vi "Periodic Tasks V.3.0.vi"(8 "error in":errorcluster) -> ()   [LabVIEW 2017]
doc: "This VI runs in parallel to other tasks. It can contain as many user-defined periodic loops as you need. These can carry out PID or other sorts of timed response."
uses:
  <vilib>/Rock Robotics/WPI/Solenoid/WPI_SolenoidValue.ctl
  <vilib>/Rock Robotics/WPI/DriverStation/WPI_DriverStationRobotMode2.ctl
  Public/Documents/Cross The Road Electronics/Phoenix-LabVIEW/Motor Controller/Get/CTRE_Phoenix_MotorController_GetQuadratureData.vi
  <vilib>/Rock Robotics/Network Tables/NT Read Boolean.vi
  Robot Global Data V.3.0.vi
  <vilib>/Rock Robotics/WPI/Utilities/WPI_GetSetVariantRefNum.vi
  <vilib>/addons/control/pid/pid.llb/PID (DBL).vi
  <vilib>/Rock Robotics/WPI/Solenoid/WPI_SolenoidSetEnum.vi
  <vilib>/Rock Robotics/WPI/RobotDrive/WPI_RobotDriveArcadeDrive_Standard(NoSaturation).vi
  <vilib>/addons/control/pid/NI_PID_pid.lvlib
panel:
  out "Right Intake Motor":dbl
  out "Left Intake Motor":dbl
  out "Read Drive Run Speed":dbl
  out "Collector and Drive Loop Run Speed":dbl
  out "Waveform Chart":T1(graph)
  in  "output range":cluster{"output high":dbl, "output low":dbl}={"output high"=100.0, "output low"=-100.0} {"output low" format="%.2f"; "output high" format="%.2f"}
  in  "PID gains":T2={"proportional gain (Kc)"=1.0, "integral time (Ti, min)"=0.01, "derivative time (Td, min)"=0.0}
  out "Compressor Run Speed":dbl
  out "Error Loop Run Speed":dbl
  out "Right Dart Run Speed":dbl
  out "Left Dart Run Speed":dbl
  out "Read Stuff Run Speed":dbl
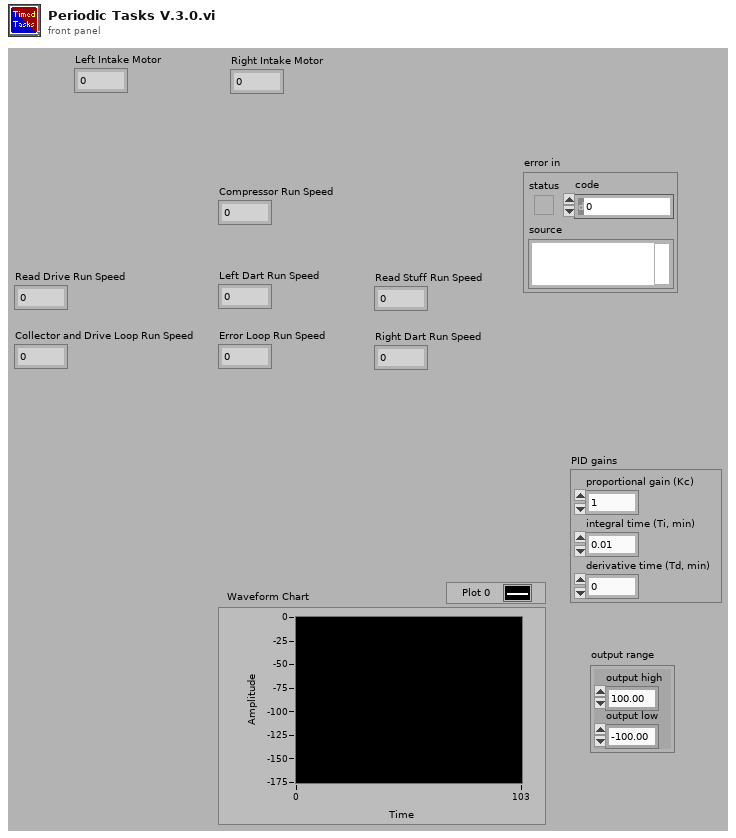
[diagram p1: front panel]
types:
  T1 = cluster{"Collector Angle Motor Wanted Angle":dbl, "Collector Angle Motor Actual Angle":dbl}
  T2 = cluster{"proportional gain (Kc)":dbl, "integral time (Ti, min)":dbl, "derivative time (Td, min)":dbl}
  T3 = cluster{"Pot. Voltage":dbl[], "Corresponding Inches":dbl[]}
  T4 = typedef "WPI_RobotDriveDevRef.ctl" = cluster{"DevStatus":errorcluster, "Motors[]":T5[], "Square Inputs":bool, "Max Output":dbl}
  T5 = typedef "WPI_MotorControlDeviceRef.ctl" = cluster{"DeviceStatus":errorcluster, "Type":T6, "PWM":cluster{"PWM Channel":T7, "DeadBand":T8}, "CAN":cluster{"Device Number":u8, "SetOutput VI Ref":variant, "GetOutput VI Ref":variant, "Enable VI Ref":variant, "Disable VI Ref":variant, "Data":variant}, "Invert":bool, "DIO PWM":cluster{"PWM \"Enable\" Channel":T7, "DIOChannel":T9, "PWM Rate":dbl}}
  T6 = typedef "WPI_MotorControlType.ctl" = enum16{"PWM", "CAN", "DIO PWM"}
  T7 = typedef "FPGA_DIOPWMChannel.ctl" = enum8{"PWM 0", "PWM 1", "PWM 2", "PWM 3", "PWM 4", "PWM 5", "PWM 6", "PWM 7", "PWM 8", "PWM 9", "PWM MXP 0", "PWM MXP 1", "PWM MXP 2", "PWM MXP 3", "PWM MXP 4", "PWM MXP 5", "PWM MXP 6", "PWM MXP 7", "PWM MXP 8", "PWM MXP 9", "Invalid"}
  T8 = typedef "WPI_PWMDeadband.ctl" = cluster{"Name":string, "maxPositivePwm":i32, "minPositivePwm":i32, "centerPwm":i32, "maxNegativePwm":i32, "minNegativePwm":i32, "angularRange":u16}
  T9 = typedef "FPGA_DIOChannel.ctl" = enum8{"DIO 0", "DIO 1", "DIO 2", "DIO 3", "DIO 4", "DIO 5", "DIO 6", "DIO 7", "DIO 8", "DIO 9", "DIO MXP 0", "DIO MXP 1", "DIO MXP 2", "DIO MXP 3", "DIO MXP 4", "DIO MXP 5", "DIO MXP 6", "DIO MXP 7", "DIO MXP 8", "DIO MXP 9", "DIO MXP 10", "DIO MXP 11", "DIO MXP 12", "DIO MXP 13", "DIO MXP 14", "DIO MXP 15", "SPI Port CS1", "SPI Port CS2", "SPI Port CS3", "SPI Port MISO", "SPI Port MOSI", "Invalid"}
  T10 = typedef "WPI_PotentiometerDevRef.ctl" = cluster{"DevStatus":errorcluster, "Analog Channel":T11, "Invert Output":bool}
  T11 = typedef "FPGA_AIChannel.ctl" = enum8{"AI 0", "AI 1", "AI 2", "AI 3", "AI MXP 0", "AI MXP 1", "AI MXP 2", "AI MXP 3", "Invalid"}
  T12 = typedef "WPI_CompressorDevRef.ctl" = cluster{"DevStatus":errorcluster, "Pneumatics Control Module":u8}
  T13 = typedef "WPI_SolenoidDevRef.ctl" = cluster{"DevStatus":errorcluster, "Pneumatics Control Module":u8, "Forward Solenoid Channel":T14, "Reverse Solenoid Channel":T14}
  T14 = typedef "WPI_SolenoidChannel.ctl" = enum8{"Solenoid 0", "Solenoid 1", "Solenoid 2", "Solenoid 3", "Solenoid 4", "Solenoid 5", "Solenoid 6", "Solenoid 7", "Invalid"}
  T15 = typedef "WPI_DriverStationRobotMode2.ctl" = enum16{"Autonomous Disabled", "Autonomous Enabled", "Teleop Disabled", "Teleop Enabled", "Disconnected", "Finish", "Test Disabled", "Test Enabled", "Emergency Stopped"}
  T16 = typedef "WPI_SolenoidValue.ctl" = enum16{"Off", "On", "Forward", "Reverse"}
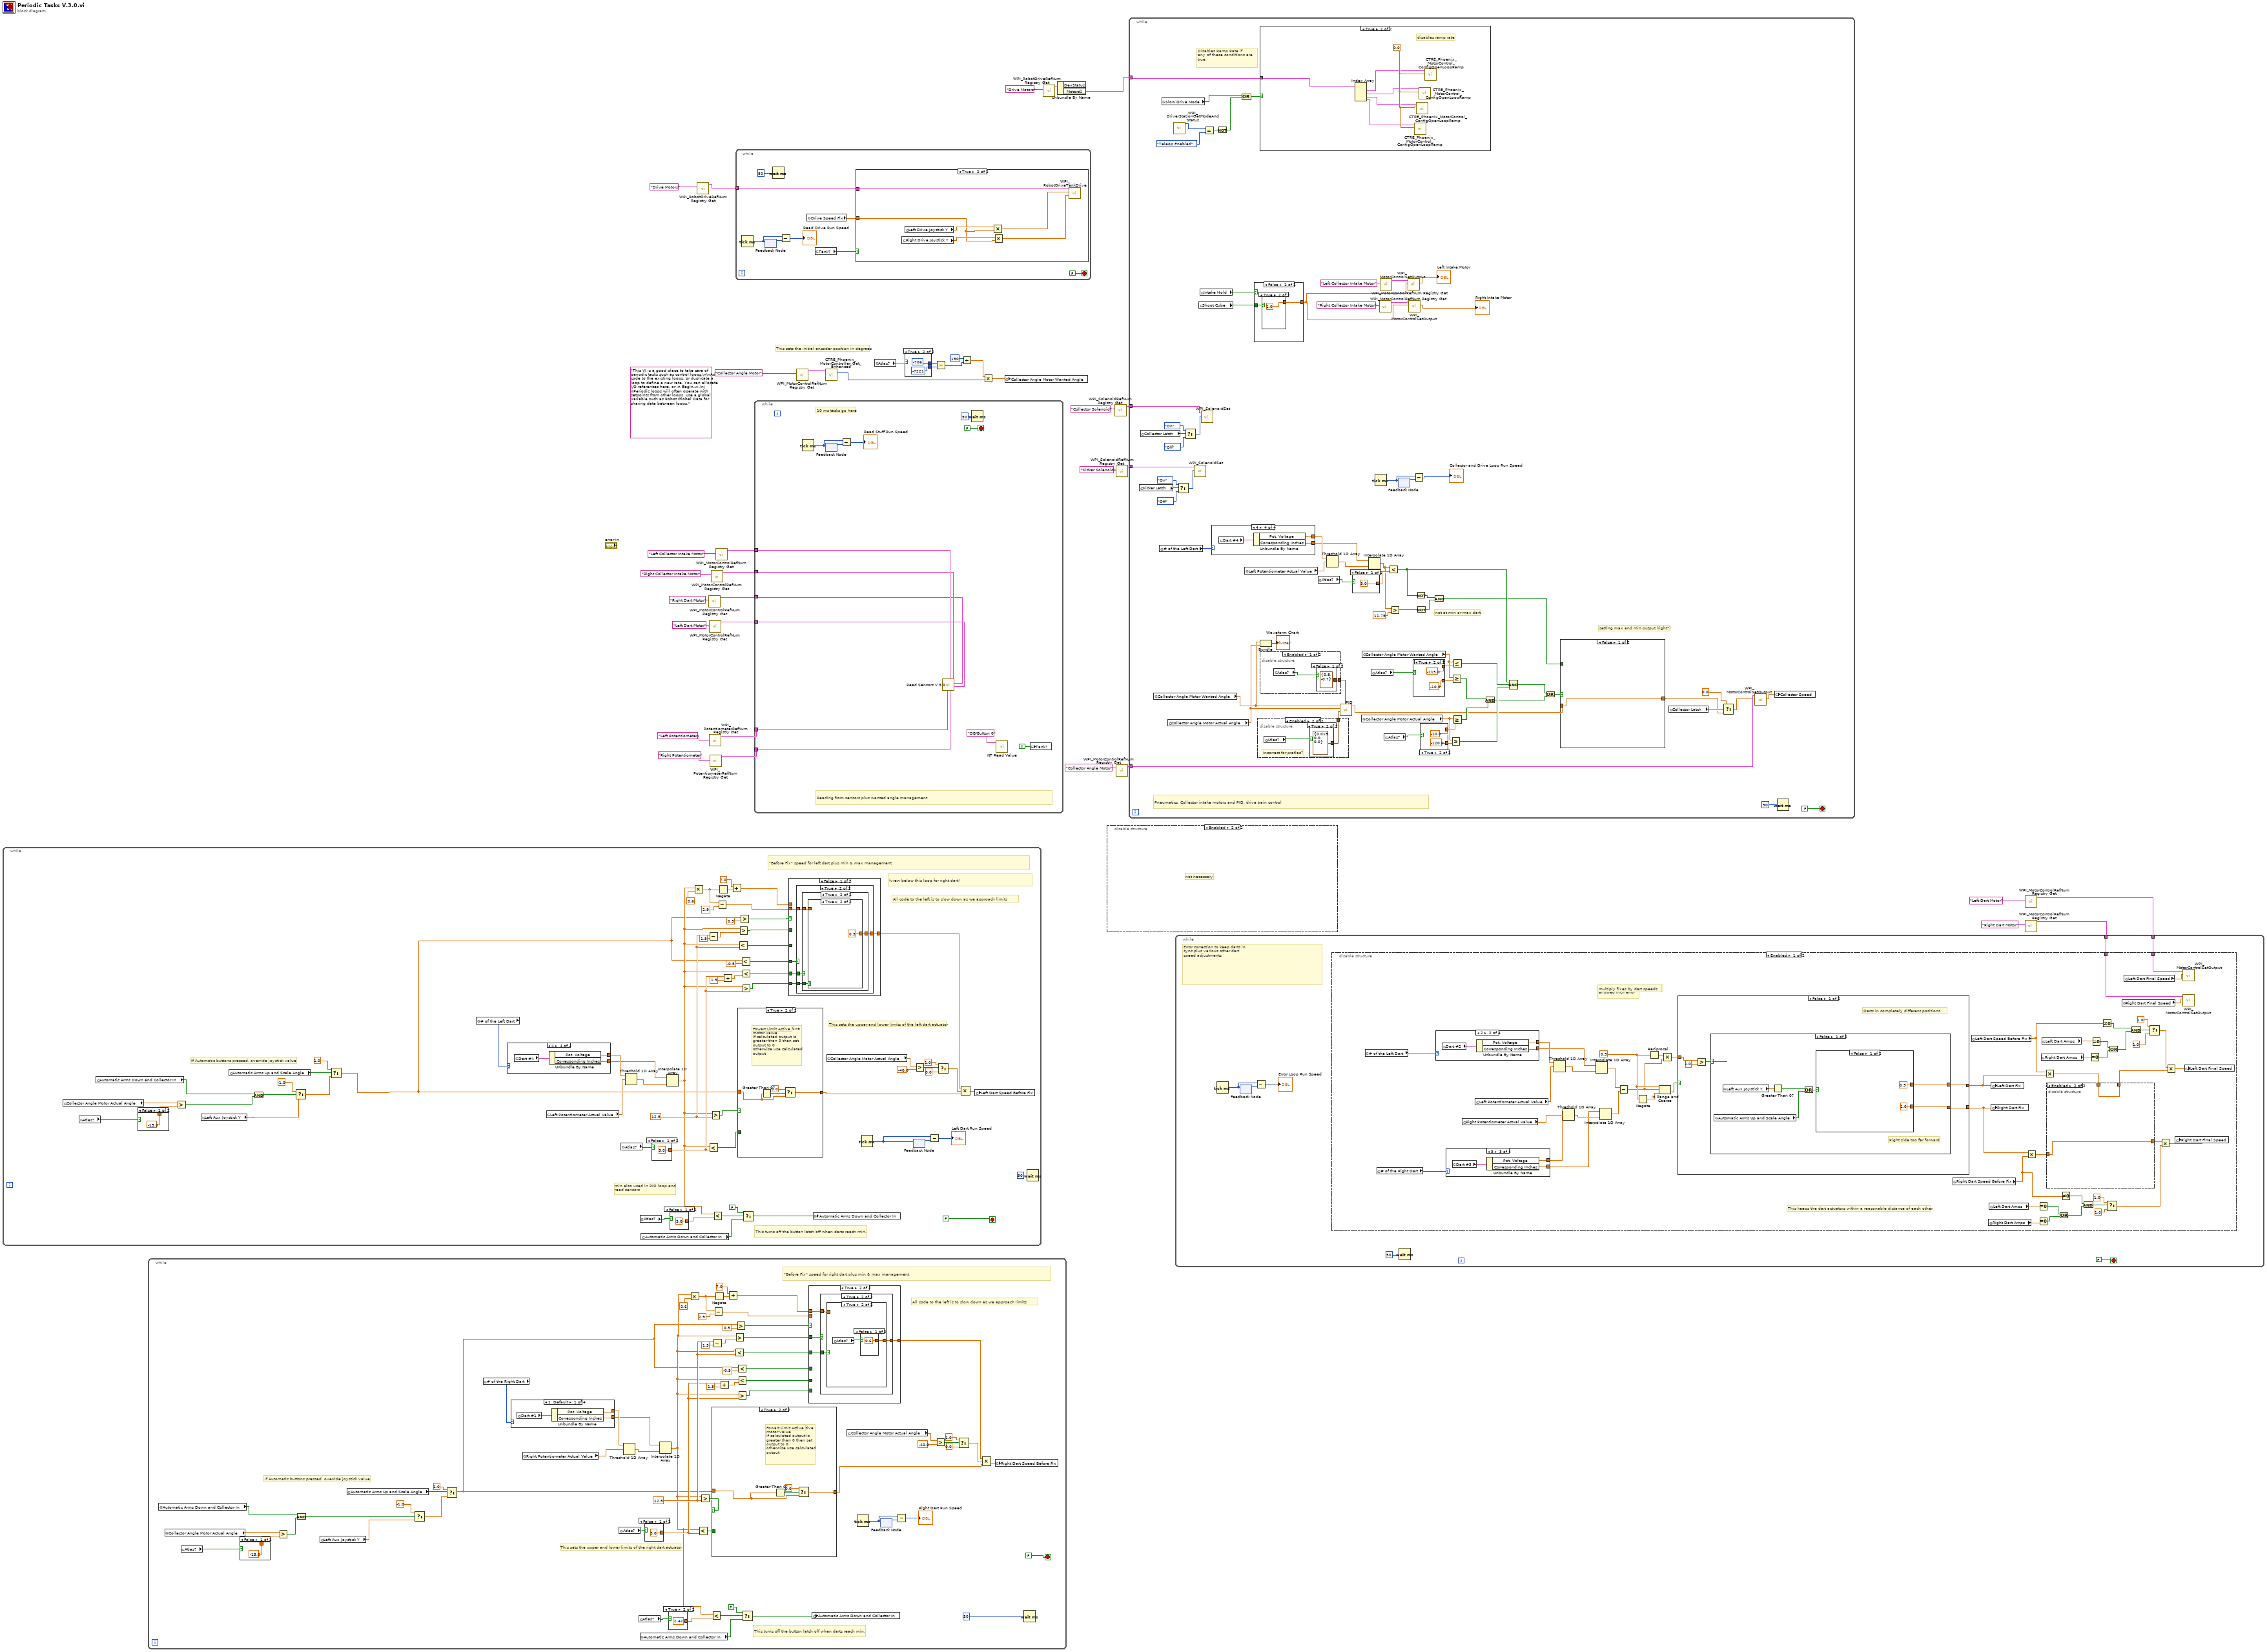
[diagram p0: block diagram]
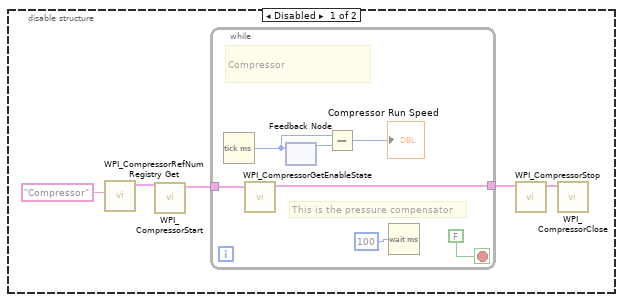
[diagram p2: hidden frame]
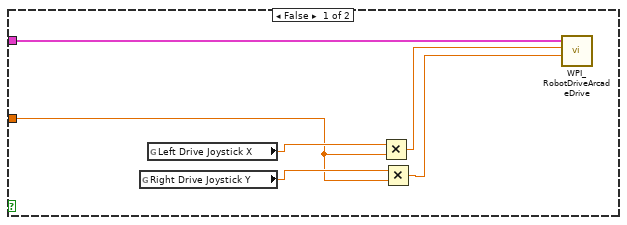
[diagram p3: hidden frame]
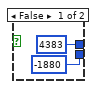
[diagram p4: hidden frame]
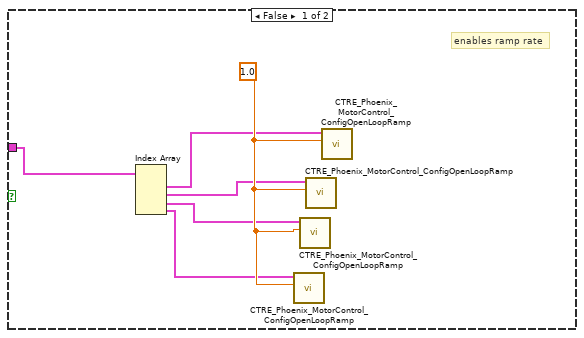
[diagram p5: hidden frame]
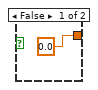
[diagram p6: hidden frame]
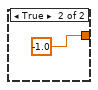
[diagram p7: hidden frame]
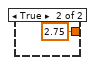
[diagram p8: hidden frame]
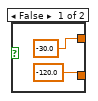
[diagram p9: hidden frame]
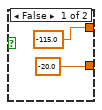
[diagram p10: hidden frame]
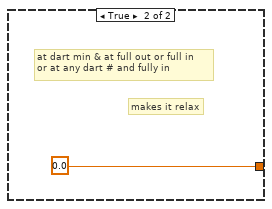
[diagram p11: hidden frame]
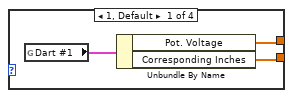
[diagram p12: hidden frame]
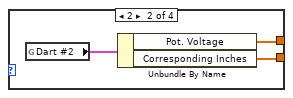
[diagram p13: hidden frame]
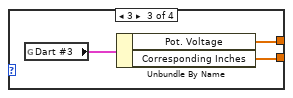
[diagram p14: hidden frame]
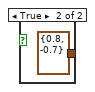
[diagram p15: hidden frame]
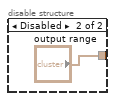
[diagram p16: hidden frame]
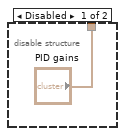
[diagram p17: hidden frame]
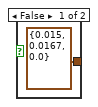
[diagram p18: hidden frame]
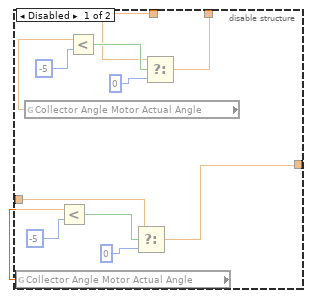
[diagram p19: hidden frame]
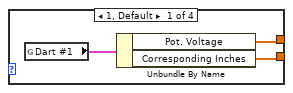
[diagram p20: hidden frame]
diagram:
  (unwired) "This VI is a good place to take care of periodic tasks such as control loops.\n\nAdd code to the existing loops, or duplicate a loop to define a new rate. You can allocate I/O references here, or in Begin.vi.\n\nPeriodic loops will often operate with setpoints from other loops. Use a global variable such as Robot Global Data for sharing data between loops."
  # "This sets the initial encoder position in degrees"
  n1 = while {
    stop <- FALSE stop-if-true
    w72 = 12.5 ("x")
    # "min also used in PID loop and \nread sensors"
    # "This turns off the button latch off when darts reach min."
    # "If Automatic buttons pressed, override joystick value"
    # "(view below this loop for right dart)"
    # "\"Before Fix\" speed for left dart plus min & max management"
    # "All code to the left is to slow down as we approach limits"
    # "This sets the upper and lower limits of the left dart actuator"
    n2 = global read "Robot Global Data V.3.0.vi" "Collector Angle Motor Actual Angle"() -> (w51:dbl)
    n3 = global read "Robot Global Data V.3.0.vi" "Atlas?"() -> (w49:bool)
    n4 = global read "Robot Global Data V.3.0.vi" "Automatic Arms Down and Collector In"() -> (w47:bool)
    n5 = case shown="False" w49 {
      tunnel: [-15.0 -35.0] -> w50
      frame False {
      }
      frame True {
      }
    }
    n6 = Greater?(x=w51, y=w50) -> (0:w46:bool)
    n7 = global read "Robot Global Data V.3.0.vi" "Left Aux Joystick Y"() -> (w52:dbl)
    n8 = global read "Robot Global Data V.3.0.vi" "Automatic Arms Up and Scale Angle"() -> (w57:bool)
    n9 = And(x=w47, y=w46) -> (x .and. y?=w48:bool)
    n10 = Select(t=-1.0, s=w48, f=w52) -> (s? t:f=w53:dbl)
    n11 = Select(t=1.0, s=w57, f=w53) -> (s? t:f=w38:dbl)
    n12 = global read "Robot Global Data V.3.0.vi" "# of the Left Dart"() -> (w91:i32)
    n13 = case shown="4" w91 {
      tunnel: [w136 w139 w142 w145] -> w93
      tunnel: [w135 w138 w141 w144] -> w92
      frame 1, Default {
        n14 = global read "Robot Global Data V.3.0.vi" "Dart #1"() -> (w137:T3)
        n15 = Unbundle By Name(w137) -> ("Pot. Voltage"=w136:dbl[], "Corresponding Inches"=w135:dbl[])
      }
      frame 2 {
        n16 = global read "Robot Global Data V.3.0.vi" "Dart #2"() -> (w140:T3)
        n17 = Unbundle By Name(w140) -> ("Pot. Voltage"=w139:dbl[], "Corresponding Inches"=w138:dbl[])
      }
      frame 3 {
        n18 = global read "Robot Global Data V.3.0.vi" "Dart #3"() -> (w143:T3)
        n19 = Unbundle By Name(w143) -> ("Pot. Voltage"=w142:dbl[], "Corresponding Inches"=w141:dbl[])
      }
      frame 4 {
        n20 = global read "Robot Global Data V.3.0.vi" "Dart #4"() -> (w146:T3)
        n21 = Unbundle By Name(w146) -> ("Pot. Voltage"=w145:dbl[], "Corresponding Inches"=w144:dbl[])
      }
    }
    n22 = global read "Robot Global Data V.3.0.vi" "Left Potentiometer Actual Value"() -> (w94:dbl)
    n23 = global read "Robot Global Data V.3.0.vi" "Atlas?"() -> (w55:bool)
    n24 = Threshold 1D Array(2:w94, 3:w93) -> (0:w95:dbl)  [unwired: 1 in]
    n25 = global read "Robot Global Data V.3.0.vi" "Atlas?"() -> (w45:bool)
    n26 = global read "Robot Global Data V.3.0.vi" "Automatic Arms Down and Collector In"() -> (w40:bool)
    n27 = case shown="False" w55 {
      tunnel: [3.0 ("x") 2.45 ("x")] -> w68
      frame False {
      }
      frame True {
      }
    }
    n28 = Interpolate 1D Array(1:w95, 2:w92) -> (0:w39:dbl)
    n29 = case shown="False" w45 {
      tunnel: [3.0 ("x") 2.42 ("x")] -> w44
      frame False {
      }
      frame True {
      }
    }
    n30 = Multiply(x=w39, y=0.6) -> (x*y=w82:dbl)
    n31 = Subtract(x=w72, y=1.5) -> (x-y=w70:dbl)
    n32 = Less?(x=w39, y=w68) -> (x < y?=w96:bool)
    n33 = Greater?(x=w39, y=w72) -> (0:w97:bool)
    n34 = Less?(x=w39, y=w44) -> (x < y?=w43:bool)
    n35 = Subtract(x=w82, y=2.9) -> (x-y=w73:dbl)
    n36 = Negate(x=w82) -> (-x=w84:dbl)
    n37 = Add(x=w68, y=1.5) -> (x+y=w69:dbl)
    n38 = Add(x=7.0, y=w84) -> (x+y=w77:dbl)
    n39 = Less?(x=w39, y=w72) -> (x < y?=w78:bool)
    n40 = Greater?(x=w39, y=w70) -> (0:w79:bool)
    n41 = case shown="True" w97 {
      tunnel: [w149 w157] -> w89
      tunnel: w38 -> [w148 w155]
      tunnel: w96 -> [w147 _]
      frame False {
        n42 = case shown="False" w147 {
          tunnel: [w150 w152] -> w149
          tunnel: w148 -> [w150 w151]
          frame False {
            # "Use calculate\nvalue"
            # "No Limits Active"
          }
          frame True {
            # "Do not allow a negitive\nmotor value\nIf calculated output is\nless than 0 then set\noutput to 0\notherwise use calculated\noutput"
            # "Back Limit Active"
            n43 = Less Than 0?(x=w151) -> (x < 0?=w154:bool)
            n44 = Select(t=0.0, s=w154, f=w151) -> (s? t:f=w152:dbl)
          }
        }
      }
      frame True {
        # "Do not allow a positive\nmotor value\nIf calculated output is\ngreater than 0 then set\noutput to 0\notherwise use calculated\noutput"
        # "Fowart Limit Active"
        n45 = Greater Than 0?(x=w155) -> (x > 0?=w158:bool)
        n46 = Select(t=0.0, s=w158, f=w155) -> (s? t:f=w157:dbl)
      }
    }
    n47 = Greater?(x=w38, y=0.5) -> (0:w80:bool)
    n48 = Less?(x=w38, y=-0.5) -> (x < y?=w76:bool)
    n49 = Less?(x=w39, y=w69) -> (x < y?=w75:bool)
    n50 = Greater?(x=w39, y=w68) -> (0:w74:bool)
    n51 = Select(t=FALSE, s=w43, f=w40) -> (s? t:f=w42:bool)
    n52 = case shown="False" w80 {
      tunnel: w79 -> [_ w125]
      tunnel: w78 -> [_ w124]
      tunnel: w77 -> [_ w123]
      tunnel: [w109 w122] -> w58
      tunnel: w76 -> [w110 _]
      tunnel: w75 -> [w108 _]
      tunnel: w74 -> [w107 _]
      tunnel: w73 -> [w106 _]
      frame False {
        n53 = case shown="True" w110 {
          tunnel: [1.0 w114] -> w109
          tunnel: w108 -> [_ w115]
          tunnel: w107 -> [_ w113]
          tunnel: w106 -> [_ w112]
          frame False {
          }
          frame True {
            n54 = case shown="True" w115 {
              tunnel: [1.0 w118] -> w114
              tunnel: w113 -> [_ w119]
              tunnel: w112 -> [_ w117]
              frame False {
              }
              frame True {
                n55 = case shown="True" w119 {
                  tunnel: [0.0 0.3] -> w118
                  tunnel: w117 -> [_ _]
                  frame False {
                  }
                  frame True {
                  }
                }
              }
            }
          }
        }
      }
      frame True {
        n56 = case shown="True" w125 {
          tunnel: w124 -> [_ w129]
          tunnel: w123 -> [_ w128]
          tunnel: [1.0 w127] -> w122
          frame False {
          }
          frame True {
            n57 = case shown="True" w129 {
              tunnel: w128 -> [_ _]
              tunnel: [0.0 w132] -> w127
              frame False {
              }
              frame True {
                n58 = global read "Robot Global Data V.3.0.vi" "Atlas?"() -> (w131:bool)
                n59 = case shown="False" w131 {
                  tunnel: [0.6 0.3] -> w132
                  frame False {
                  }
                  frame True {
                  }
                }
              }
            }
          }
        }
      }
    }
    n60 = global write "Robot Global Data V.3.0.vi" "Automatic Arms Down and Collector In"(w42) -> ()
    n61 = global read "Robot Global Data V.3.0.vi" "Collector Angle Motor Actual Angle"() -> (w64:dbl)
    n62 = Tick Count (ms)() -> (millisecond timer value=w87:u32)
    n63 = feedback #1() -> (w88:u32)  [unwired: 1 in]
    n64 = feedback-in #1(w87) -> ()
    n65 = Greater?(x=w64, y=-40.0) -> (0:w62:bool)
    n66 = Subtract(x=w87, y=w88) -> (x-y=→"Left Dart Run Speed":u32)
    n67 = Select(t=1.0, s=w62, f=0.0) -> (s? t:f=w59:dbl)
    n68 = Compound Arithmetic op=MULTIPLY(w58, w59, w89) -> (w90:dbl)
    n69 = global write "Robot Global Data V.3.0.vi" "Left Dart Speed Before Fix"(w90) -> ()
    n70 = Wait (ms)(milliseconds to wait=u32 50) -> ()  [unwired: 1 out]
  }
  n71 = while {
    stop <- FALSE stop-if-true
    w193 = 12.5 ("x")
    # "This turns off the button latch off when darts reach min."
    # "If Automatic buttons pressed, override joystick value"
    # "\"Before Fix\" speed for right dart plus min & max management"
    # "All code to the left is to slow down as we approach limits"
    # "This sets the upper and lower limits of the right dart actuator"
    n72 = global read "Robot Global Data V.3.0.vi" "Automatic Arms Down and Collector In"() -> (w170:bool)
    n73 = global read "Robot Global Data V.3.0.vi" "Collector Angle Motor Actual Angle"() -> (w173:dbl)
    n74 = global read "Robot Global Data V.3.0.vi" "Atlas?"() -> (w171:bool)
    n75 = case shown="False" w171 {
      tunnel: [-15.0 -35.0] -> w172
      frame False {
      }
      frame True {
      }
    }
    n76 = Greater?(x=w173, y=w172) -> (0:w169:bool)
    n77 = And(x=w170, y=w169) -> (x .and. y?=w168:bool)
    n78 = global read "Robot Global Data V.3.0.vi" "Left Aux Joystick Y"() -> (w175:dbl)
    n79 = global read "Robot Global Data V.3.0.vi" "Automatic Arms Up and Scale Angle"() -> (w179:bool)
    n80 = Select(t=-1.0, s=w168, f=w175) -> (s? t:f=w174:dbl)
    n81 = Select(t=1.0, s=w179, f=w174) -> (s? t:f=w159:dbl)
    n82 = global read "Robot Global Data V.3.0.vi" "# of the Right Dart"() -> (w213:i32)
    n83 = case shown="1, Default" w213 {
      tunnel: [w257 w260 w263 w266] -> w215
      tunnel: [w256 w259 w262 w265] -> w214
      frame 1, Default {
        n84 = global read "Robot Global Data V.3.0.vi" "Dart #1"() -> (w258:T3)
        n85 = Unbundle By Name(w258) -> ("Pot. Voltage"=w257:dbl[], "Corresponding Inches"=w256:dbl[])
      }
      frame 2 {
        n86 = global read "Robot Global Data V.3.0.vi" "Dart #2"() -> (w261:T3)
        n87 = Unbundle By Name(w261) -> ("Pot. Voltage"=w260:dbl[], "Corresponding Inches"=w259:dbl[])
      }
      frame 3 {
        n88 = global read "Robot Global Data V.3.0.vi" "Dart #3"() -> (w264:T3)
        n89 = Unbundle By Name(w264) -> ("Pot. Voltage"=w263:dbl[], "Corresponding Inches"=w262:dbl[])
      }
      frame 4 {
        n90 = global read "Robot Global Data V.3.0.vi" "Dart #4"() -> (w267:T3)
        n91 = Unbundle By Name(w267) -> ("Pot. Voltage"=w266:dbl[], "Corresponding Inches"=w265:dbl[])
      }
    }
    n92 = global read "Robot Global Data V.3.0.vi" "Right Potentiometer Actual Value"() -> (w216:dbl)
    n93 = global read "Robot Global Data V.3.0.vi" "Atlas?"() -> (w177:bool)
    n94 = Threshold 1D Array(2:w216, 3:w215) -> (0:w217:dbl)  [unwired: 1 in]
    n95 = global read "Robot Global Data V.3.0.vi" "Atlas?"() -> (w166:bool)
    n96 = global read "Robot Global Data V.3.0.vi" "Automatic Arms Down and Collector In"() -> (w161:bool)
    n97 = case shown="False" w177 {
      tunnel: [3.0 ("x") 2.45 ("x")] -> w190
      frame False {
      }
      frame True {
      }
    }
    n98 = Interpolate 1D Array(1:w217, 2:w214) -> (0:w160:dbl)
    n99 = case shown="True" w166 {
      tunnel: [3.0 ("x") 2.42 ("x")] -> w165
      frame False {
      }
      frame True {
      }
    }
    n100 = Multiply(x=w160, y=0.6) -> (x*y=w207:dbl)
    n101 = Less?(x=w160, y=w190) -> (x < y?=w167:bool)
    n102 = Greater?(x=w160, y=w193) -> (0:w218:bool)
    n103 = Less?(x=w160, y=w165) -> (x < y?=w164:bool)
    n104 = Subtract(x=w193, y=1.5) -> (x-y=w194:dbl)
    n105 = case shown="True" w218 {
      tunnel: [w270 w278] -> w212
      tunnel: w159 -> [w269 w276]
      tunnel: w167 -> [w268 _]
      frame False {
        n106 = case shown="True" w268 {
          tunnel: [w271 w273] -> w270
          tunnel: w269 -> [w271 w272]
          frame False {
            # "Use calculate\nvalue"
            # "No Limits Active"
          }
          frame True {
            # "Do not allow a negitive\nmotor value\nIf calculated output is\nless than 0 then set\noutput to 0\notherwise use calculated\noutput"
            # "Back Limit Active"
            n107 = Less Than 0?(x=w272) -> (x < 0?=w275:bool)
            n108 = Select(t=0.0, s=w275, f=w272) -> (s? t:f=w273:dbl)
          }
        }
      }
      frame True {
        # "Do not allow a positive\nmotor value\nIf calculated output is\ngreater than 0 then set\noutput to 0\notherwise use calculated\noutput"
        # "Fowart Limit Active"
        n109 = Greater Than 0?(x=w276) -> (x > 0?=w279:bool)
        n110 = Select(t=0.0, s=w279, f=w276) -> (s? t:f=w278:dbl)
      }
    }
    n111 = Subtract(x=w207, y=2.9) -> (x-y=w195:dbl)
    n112 = Negate(x=w207) -> (-x=w209:dbl)
    n113 = Add(x=w190, y=1.5) -> (x+y=w191:dbl)
    n114 = Add(x=7.0, y=w209) -> (x+y=w199:dbl)
    n115 = Less?(x=w160, y=w193) -> (x < y?=w200:bool)
    n116 = Greater?(x=w160, y=w194) -> (0:w201:bool)
    n117 = Greater?(x=w159, y=0.5) -> (0:w202:bool)
    n118 = Less?(x=w159, y=-0.5) -> (x < y?=w198:bool)
    n119 = Less?(x=w160, y=w191) -> (x < y?=w197:bool)
    n120 = Greater?(x=w160, y=w190) -> (0:w196:bool)
    n121 = Select(t=FALSE, s=w164, f=w161) -> (s? t:f=w163:bool)
    n122 = case shown="True" w202 {
      tunnel: w201 -> [_ w246]
      tunnel: w200 -> [_ w245]
      tunnel: w199 -> [_ w244]
      tunnel: [w230 w243] -> w180
      tunnel: w198 -> [w231 _]
      tunnel: w197 -> [w229 _]
      tunnel: w196 -> [w228 _]
      tunnel: w195 -> [w227 _]
      frame False {
        n123 = case shown="True" w231 {
          tunnel: [1.0 w235] -> w230
          tunnel: w229 -> [_ w236]
          tunnel: w228 -> [_ w234]
          tunnel: w227 -> [_ w233]
          frame False {
          }
          frame True {
            n124 = case shown="True" w236 {
              tunnel: [1.0 w239] -> w235
              tunnel: w234 -> [_ w240]
              tunnel: w233 -> [_ w238]
              frame False {
              }
              frame True {
                n125 = case shown="True" w240 {
                  tunnel: [0.0 0.3] -> w239
                  tunnel: w238 -> [_ _]
                  frame False {
                  }
                  frame True {
                  }
                }
              }
            }
          }
        }
      }
      frame True {
        n126 = case shown="True" w246 {
          tunnel: w245 -> [_ w250]
          tunnel: w244 -> [_ w249]
          tunnel: [1.0 w248] -> w243
          frame False {
          }
          frame True {
            n127 = case shown="True" w250 {
              tunnel: w249 -> [_ _]
              tunnel: [0.0 w252] -> w248
              frame False {
              }
              frame True {
                n128 = global read "Robot Global Data V.3.0.vi" "Atlas?"() -> (w253:bool)
                n129 = case shown="False" w253 {
                  tunnel: [0.6 0.3] -> w252
                  frame False {
                  }
                  frame True {
                  }
                }
              }
            }
          }
        }
      }
    }
    n130 = global write "Robot Global Data V.3.0.vi" "Automatic Arms Down and Collector In"(w163) -> ()
    n131 = global read "Robot Global Data V.3.0.vi" "Collector Angle Motor Actual Angle"() -> (w186:dbl)
    n132 = Tick Count (ms)() -> (millisecond timer value=w204:u32)
    n133 = feedback #2() -> (w205:u32)  [unwired: 1 in]
    n134 = feedback-in #2(w204) -> ()
    n135 = Subtract(x=w204, y=w205) -> (x-y=→"Right Dart Run Speed":u32)
    n136 = Greater?(x=w186, y=-40.0) -> (0:w184:bool)
    n137 = Select(t=1.0, s=w184, f=0.0) -> (s? t:f=w181:dbl)
    n138 = Compound Arithmetic op=MULTIPLY(w180, w181, w212) -> (w211:dbl)
    n139 = global write "Robot Global Data V.3.0.vi" "Right Dart Speed Before Fix"(w211) -> ()
    n140 = Wait (ms)(milliseconds to wait=u32 50) -> ()  [unwired: 1 out]
  }
  n141 = call <vilib>:"WPI_RobotDriveRefNum Registry Get.vi"("refnum name"="Drive Motors") -> ("RobotDriveDevRef"=w1:T4)  [unwired: 9 in, 1 out]
  n142 = call <vilib>:"WPI_MotorControlRefNum Registry Get.vi"("refnum name"="Right Dart Motor") -> ("MotorControlDevRef"=w25:T5)  [unwired: 9 in, 1 out]
  n143 = call <vilib>:"WPI_MotorControlRefNum Registry Get.vi"("refnum name"="Left Dart Motor") -> ("MotorControlDevRef"=w24:T5)  [unwired: 9 in, 1 out]
  n144 = call <vilib>:"WPI_PotentiometerRefNum Registry Get.vi"("refnum name"="Left Potentiometer") -> ("PotDevRef"=w34:T10)  [unwired: 9 in, 1 out]
  n145 = call <vilib>:"WPI_PotentiometerRefNum Registry Get.vi"("refnum name"="Right Potentiometer") -> ("PotDevRef"=w37:T10)  [unwired: 9 in, 1 out]
  n146 = call <vilib>:"WPI_MotorControlRefNum Registry Get.vi"("refnum name"="Right Collector Intake Motor") -> ("MotorControlDevRef"=w30:T5)  [unwired: 9 in, 1 out]
  n147 = call <vilib>:"WPI_MotorControlRefNum Registry Get.vi"("refnum name"="Left Collector Intake Motor") -> ("MotorControlDevRef"=w31:T5)  [unwired: 9 in, 1 out]
  n148 = while {
    tunnel: w1 -> [w285]
    stop <- FALSE stop-if-true
    n149 = Tick Count (ms)() -> (millisecond timer value=w281:u32)
    n150 = feedback #3() -> (w282:u32)  [unwired: 1 in]
    n151 = feedback-in #3(w281) -> ()
    n152 = Wait (ms)(milliseconds to wait=50) -> ()  [unwired: 1 out]
    n153 = Subtract(x=w281, y=w282) -> (x-y=→"Read Drive Run Speed":u32)
    n154 = global read "Robot Global Data V.3.0.vi" "Drive Speed Fix"() -> (w286:dbl)
    n155 = global read "Robot Global Data V.3.0.vi" "Tank?"() -> (w287:bool)
    n156 = case shown="True" w287 {
      tunnel: w286 -> [w288 w295]
      tunnel: w285 -> [w291 w294]
      frame False {
        n157 = global read "Robot Global Data V.3.0.vi" "Right Drive Joystick Y"() -> (w292:dbl)
        n158 = global read "Robot Global Data V.3.0.vi" "Left Drive Joystick X"() -> (w293:dbl)
        n159 = Multiply(x=w293, y=w288) -> (x*y=w290:dbl)
        n160 = Multiply(x=w292, y=w288) -> (x*y=w289:dbl)
        n161 = call-poly <vilib>:"WPI_RobotDriveArcadeDrive.vi"("Y axis value"=w289, "X axis value"=w290, "RobotDriveDevRef"=w291) -> ()  [unwired: 6 in, 3 out]
      }
      frame True {
        n162 = global read "Robot Global Data V.3.0.vi" "Right Drive Joystick Y"() -> (w296:dbl)
        n163 = global read "Robot Global Data V.3.0.vi" "Left Drive Joystick Y"() -> (w297:dbl)
        n164 = Multiply(x=w297, y=w295) -> (x*y=w299:dbl)
        n165 = Multiply(x=w296, y=w295) -> (x*y=w298:dbl)
        n166 = call <vilib>:"WPI_RobotDriveTankDrive.vi"("Right axis value"=w298, "Left axis value"=w299, "RobotDriveDevRef"=w294) -> ()  [unwired: 6 in, 3 out]
      }
    }
  }
  n167 = while {
    tunnel: w37 -> [w309]
    tunnel: w34 -> [w310]
    tunnel: w31 -> [w307]
    tunnel: w30 -> [w306]
    tunnel: w25 -> [w305]
    tunnel: w24 -> [w304]
    stop <- FALSE stop-if-true
    # "Reading from sensors plus wanted angle management"
    # "10 ms tasks go here"
    n168 = Tick Count (ms)() -> (millisecond timer value=w302:u32)
    n169 = feedback #4() -> (w303:u32)  [unwired: 1 in]
    n170 = feedback-in #4(w302) -> ()
    n171 = Subtract(x=w302, y=w303) -> (x-y=→"Read Stuff Run Speed":u32)
    n172 = call "Read Sensors V.3.0.vi"("Left Dart Motor"=w304, "Right Dart Motor"=w305, "Right Collector Intake Motor"=w306, "Right Pot."=w309, "Left Collector Intake Motor"=w307, "Left Pot."=w310) -> ()  [unwired: 6 in]
    n173 = Wait (ms)(milliseconds to wait=u32 50) -> ()  [unwired: 1 out]
    n174 = call-poly <vilib>:"NT Read Value.vi"("Name"="DB/Button 0") -> ()  [unwired: 9 in, 2 out]
    n175 = global write "Robot Global Data V.3.0.vi" "Tank?"(TRUE) -> ()
  }
  n176 = call <vilib>:"WPI_MotorControlRefNum Registry Get.vi"("refnum name"="Collector Angle Motor") -> ("MotorControlDevRef"=w29:T5)  [unwired: 9 in, 1 out]
  n177 = call-poly "CTRE_Phoenix_MotorController_Get_Enhanced.vi"("PhoenixMotorControlDevRef"=w29) -> ("Quadrature Position"=w20:i32)  [unwired: 11 in, 3 out]
  n178 = global read "Robot Global Data V.3.0.vi" "Atlas?"() -> (w17:bool)
  n179 = case shown="True" w17 {
    tunnel: [4383 -706] -> w19
    tunnel: [-1880 -7221] -> w18
    frame False {
    }
    frame True {
    }
  }
  n180 = Subtract(x=w19, y=w18) -> (x-y=w16:i32)
  n181 = Divide(x=180, y=w16) -> (x/y=w22:dbl)
  n182 = Multiply(x=w22, y=w20) -> (x*y=w21:dbl)
  n183 = global write "Robot Global Data V.3.0.vi" "Collector Angle Motor Wanted Angle"(w21) -> ()
  n184 = call <vilib>:"WPI_RobotDriveRefNum Registry Get.vi"("refnum name"="Drive Motors") -> ("RobotDriveDevRef"=w15:T4)  [unwired: 9 in, 1 out]
  n185 = Unbundle By Name(w15) -> ("Motors[]"=w13:T5[])  [unwired: 1 out]
  n186 = disable-structure shown="Enabled" {
    frame Disabled {
      n187 = call <vilib>:"WPI_CompressorRefNum Registry Get.vi"("refnum name"="Compressor") -> ("CompressorDevRef"=w318:T12)  [unwired: 9 in, 1 out]
      n188 = call <vilib>:"WPI_CompressorStart.vi"("CompressorDevRef"=w318) -> ("CompressorDevRef"=w317:T12)  [unwired: 9 in, 1 out]
      n189 = while {
        tunnel: [w326] -> w321
        tunnel: w317 -> [w325]
        stop <- FALSE stop-if-true
        # "Compressor"
        # "This is the pressure compensator"
        n190 = Tick Count (ms)() -> (millisecond timer value=w323:u32)
        n191 = call <vilib>:"WPI_CompressorGetEnableState.vi"("CompressorDevRef"=w325) -> ("CompressorDevRef"=w326:T12)  [unwired: 7 in, 3 out]
        n192 = feedback #5() -> (w324:u32)  [unwired: 1 in]
        n193 = feedback-in #5(w323) -> ()
        n194 = Subtract(x=w323, y=w324) -> (x-y=→"Compressor Run Speed":u32)
        n195 = Wait (ms)(milliseconds to wait=100) -> ()  [unwired: 1 out]
      }
      n196 = call <vilib>:"WPI_CompressorStop.vi"("CompressorDevRef"=w321) -> ("CompressorDevRef"=w320:T12)  [unwired: 9 in, 1 out]
      n197 = call <vilib>:"WPI_CompressorClose.vi"("CompressorDevRef"=w320) -> ()  [unwired: 10 in, 1 out]
    }
    frame Enabled {
      # "not necessary"
    }
  }
  n198 = call <vilib>:"WPI_SolenoidRefNum Registry Get.vi"("refnum name"="Collector Solenoid") -> ("SolenoidDevRef"=w9:T13)  [unwired: 9 in, 1 out]
  n199 = call <vilib>:"WPI_SolenoidRefNum Registry Get.vi"("refnum name"="Kicker Solenoid") -> ("SolenoidDevRef"=w11:T13)  [unwired: 9 in, 1 out]
  n200 = call <vilib>:"WPI_MotorControlRefNum Registry Get.vi"("refnum name"="Collector Angle Motor") -> ("MotorControlDevRef"=w7:T5)  [unwired: 9 in, 1 out]
  n201 = while {
    tunnel: w13 -> [w398]
    tunnel: w11 -> [w397]
    tunnel: w9 -> [w396]
    tunnel: w7 -> [w395]
    stop <- FALSE stop-if-true
    # "Disables Ramp Rate if\nany of these conditions are\ntrue"
    # "not at min or max dart"
    # "setting max and min output (right?)"
    # "Pneumatics, Collector intake motors and PID, drive train control"
    n202 = global read "Robot Global Data V.3.0.vi" "Kicker Latch"() -> (w387:bool)
    n203 = global read "Robot Global Data V.3.0.vi" "Collector Latch"() -> (w391:bool)
    n204 = global read "Robot Global Data V.3.0.vi" "Collector Angle Motor Wanted Angle"() -> (w379:dbl)
    n205 = global read "Robot Global Data V.3.0.vi" "# of the Left Dart"() -> (w361:i32)
    n206 = global read "Robot Global Data V.3.0.vi" "Slow Drive Mode"() -> (w332:bool)
    n207 = global read "Robot Global Data V.3.0.vi" "Collector Angle Motor Actual Angle"() -> (w378:dbl)
    n208 = call <vilib>:"WPI_DriverStationGetModeAndStatus.vi"() -> ("Robot Mode"=w334:T15)  [unwired: 10 in, 1 out]
    n209 = Select(t=WPI_SolenoidValue."On" ("Value"), s=w387, f=WPI_SolenoidValue."Off" ("Value")) -> (s? t:f=w384:T16)
    n210 = Select(t=WPI_SolenoidValue."On" ("Value"), s=w391, f=WPI_SolenoidValue."Off" ("Value")) -> (s? t:f=w388:T16)
    n211 = call-poly <vilib>:"WPI_SolenoidSet.vi"("Value"=w384, "SolenoidDevRef"=w397) -> ()  [unwired: 8 in, 2 out]
    n212 = global read "Robot Global Data V.3.0.vi" "Shoot Cube"() -> (w337:bool)
    n213 = global read "Robot Global Data V.3.0.vi" "Intake Hold"() -> (w338:bool)
    n214 = call-poly <vilib>:"WPI_SolenoidSet.vi"("Value"=w388, "SolenoidDevRef"=w396) -> ()  [unwired: 8 in, 2 out]
    n215 = Equal?(x=w334, y=WPI_DriverStationRobotMode2."Teleop Enabled" ("Robot Mode")) -> (x = y?=w333:bool)
    n216 = case shown="4" w361 {
      tunnel: [w431 w434 w437 w440] -> w363
      tunnel: [w430 w433 w436 w439] -> w362
      frame 1, Default {
        n217 = global read "Robot Global Data V.3.0.vi" "Dart #1"() -> (w432:T3)
        n218 = Unbundle By Name(w432) -> ("Pot. Voltage"=w431:dbl[], "Corresponding Inches"=w430:dbl[])
      }
      frame 2 {
        n219 = global read "Robot Global Data V.3.0.vi" "Dart #2"() -> (w435:T3)
        n220 = Unbundle By Name(w435) -> ("Pot. Voltage"=w434:dbl[], "Corresponding Inches"=w433:dbl[])
      }
      frame 3 {
        n221 = global read "Robot Global Data V.3.0.vi" "Dart #3"() -> (w438:T3)
        n222 = Unbundle By Name(w438) -> ("Pot. Voltage"=w437:dbl[], "Corresponding Inches"=w436:dbl[])
      }
      frame 4 {
        n223 = global read "Robot Global Data V.3.0.vi" "Dart #4"() -> (w441:T3)
        n224 = Unbundle By Name(w441) -> ("Pot. Voltage"=w440:dbl[], "Corresponding Inches"=w439:dbl[])
      }
    }
    n225 = Not(x=w333) -> (.not. x?=w331:bool)
    n226 = Compound Arithmetic op=OR(w332, w331) -> (w336:bool)
    n227 = global read "Robot Global Data V.3.0.vi" "Left Potentiometer Actual Value"() -> (w364:dbl)
    n228 = case shown="False" w338 {
      tunnel: [w413 -1.0] -> w339
      tunnel: w337 -> [w414 _]
      frame False {
        n229 = case shown="True" w414 {
          tunnel: [0.0 1.0] -> w413
          frame False {
          }
          frame True {
          }
        }
      }
      frame True {
      }
    }
    n230 = disable-structure shown="Enabled" {
      disable-tunnel: ["PID gains" w449] -> w381
      frame Disabled {
      }
      frame Enabled {
        # "incorrect for pratlas?"
        n231 = global read "Robot Global Data V.3.0.vi" "Atlas?"() -> (w448:bool)
        n232 = case shown="True" w448 {
          tunnel: [T2 {"proportional gain (Kc)"=0.015, "integral time (Ti, min)"=0.0167, "derivative time (Td, min)"=0.0} ("PID gains") T2 {"proportional gain (Kc)"=0.015, "integral time (Ti, min)"=0.0, "derivative time (Td, min)"=0.0} ("PID gains")] -> w449
          frame False {
          }
          frame True {
          }
        }
      }
    }
    n233 = case shown="True" w336 {
      tunnel: w398 -> [w401 w407]
      frame False {
        w406 = 1.0
        # "enables ramp rate"
        n234 = Index Array(array=w401) -> (element #1=w405:T5, element #2=w404:T5, element #3=w403:T5, element #4=w402:T5)  [unwired: 4 in]
        n235 = call "CTRE_Phoenix_MotorControl_ConfigOpenLoopRamp.vi"("secondsFromNeutralToFull"=w406, "PhoenixMotorControlDevRef"=w402) -> ()  [unwired: 8 in, 2 out]
        n236 = call "CTRE_Phoenix_MotorControl_ConfigOpenLoopRamp.vi"("secondsFromNeutralToFull"=w406, "PhoenixMotorControlDevRef"=w403) -> ()  [unwired: 8 in, 2 out]
        n237 = call "CTRE_Phoenix_MotorControl_ConfigOpenLoopRamp.vi"("secondsFromNeutralToFull"=w406, "PhoenixMotorControlDevRef"=w404) -> ()  [unwired: 8 in, 2 out]
        n238 = call "CTRE_Phoenix_MotorControl_ConfigOpenLoopRamp.vi"("secondsFromNeutralToFull"=w406, "PhoenixMotorControlDevRef"=w405) -> ()  [unwired: 8 in, 2 out]
      }
      frame True {
        w412 = 0.0
        # "disables ramp rate"
        n239 = Index Array(array=w407) -> (element #1=w411:T5, element #2=w410:T5, element #3=w409:T5, element #4=w408:T5)  [unwired: 4 in]
        n240 = call "CTRE_Phoenix_MotorControl_ConfigOpenLoopRamp.vi"("secondsFromNeutralToFull"=w412, "PhoenixMotorControlDevRef"=w408) -> ()  [unwired: 8 in, 2 out]
        n241 = call "CTRE_Phoenix_MotorControl_ConfigOpenLoopRamp.vi"("secondsFromNeutralToFull"=w412, "PhoenixMotorControlDevRef"=w409) -> ()  [unwired: 8 in, 2 out]
        n242 = call "CTRE_Phoenix_MotorControl_ConfigOpenLoopRamp.vi"("secondsFromNeutralToFull"=w412, "PhoenixMotorControlDevRef"=w410) -> ()  [unwired: 8 in, 2 out]
        n243 = call "CTRE_Phoenix_MotorControl_ConfigOpenLoopRamp.vi"("secondsFromNeutralToFull"=w412, "PhoenixMotorControlDevRef"=w411) -> ()  [unwired: 8 in, 2 out]
      }
    }
    n244 = disable-structure shown="Enabled" {
      disable-tunnel: [w443 "output range"] -> w383
      frame Enabled {
        n245 = global read "Robot Global Data V.3.0.vi" "Atlas?"() -> (w442:bool)
        n246 = case shown="False" w442 {
          tunnel: [cluster{"output high":dbl, "output low":dbl} {"output high"=0.8, "output low"=-0.7} ("output range") cluster{"output high":dbl, "output low":dbl} {"output high"=0.8, "output low"=-0.7} ("output range")] -> w443
          frame False {
          }
          frame True {
          }
        }
      }
      frame Disabled {
      }
    }
    n247 = Bundle("Collector Angle Motor Wanted Angle"=w379, "Collector Angle Motor Actual Angle"=w378) -> (→"Waveform Chart":T1)  [unwired: 1 in]
    n248 = global read "Robot Global Data V.3.0.vi" "Atlas?"() -> (w344:bool)
    n249 = Threshold 1D Array(2:w364, 3:w363) -> (0:w365:dbl)  [unwired: 1 in]
    n250 = call-poly <vilib>:"PID.vi"("output range"=w383, "PID gains"=w381, "process variable"=w378, "setpoint"=w379) -> ("output"=w347:dbl)  [unwired: 6 in, 1 out]
    n251 = case shown="False" w344 {
      tunnel: [3.0 2.75 ("y")] -> w360
      frame False {
      }
      frame True {
      }
    }
    n252 = global read "Robot Global Data V.3.0.vi" "Collector Angle Motor Actual Angle"() -> (w376:dbl)
    n253 = global read "Robot Global Data V.3.0.vi" "Collector Angle Motor Wanted Angle"() -> (w373:dbl)
    n254 = Interpolate 1D Array(1:w365, 2:w362) -> (0:w354:dbl)
    n255 = global read "Robot Global Data V.3.0.vi" "Atlas?"() -> (w346:bool)
    n256 = Tick Count (ms)() -> (millisecond timer value=w393:u32)
    n257 = call <vilib>:"WPI_MotorControlRefNum Registry Get.vi"("refnum name"="Right Collector Intake Motor") -> ("MotorControlDevRef"=w341:T5)  [unwired: 9 in, 1 out]
    n258 = call <vilib>:"WPI_MotorControlRefNum Registry Get.vi"("refnum name"="Left Collector Intake Motor") -> ("MotorControlDevRef"=w340:T5)  [unwired: 9 in, 1 out]
    n259 = global read "Robot Global Data V.3.0.vi" "Atlas?"() -> (w345:bool)
    n260 = Less?(x=w354, y=w360) -> (x < y?=w355:bool)
    n261 = Greater?(x=w354, y=11.75) -> (0:w352:bool)
    n262 = feedback #6() -> (w394:u32)  [unwired: 1 in]
    n263 = feedback-in #6(w393) -> ()
    n264 = call <vilib>:"WPI_MotorControlSetOutput.vi"("Output"=w339, "MotorControlDevRef"=w340) -> ("Motor Output"=→"Left Intake Motor":dbl)  [unwired: 7 in, 2 out]
    n265 = call <vilib>:"WPI_MotorControlSetOutput.vi"("Output"=w339, "MotorControlDevRef"=w341) -> ("Motor Output"=→"Right Intake Motor":dbl)  [unwired: 7 in, 2 out]
    n266 = case shown="True" w346 {
      tunnel: [-20.0 ("y") -10.0 ("y")] -> w374
      tunnel: [-115.0 ("y") -115.0 ("y")] -> w372
      frame False {
      }
      frame True {
      }
    }
    n267 = Subtract(x=w393, y=w394) -> (x-y=→"Collector and Drive Loop Run Speed":u32)
    n268 = Not(x=w355) -> (.not. x?=w356:bool)
    n269 = Not(x=w352) -> (.not. x?=w351:bool)
    n270 = case shown="True" w345 {
      tunnel: [-30.0 ("y") -10.0 ("y")] -> w377
      tunnel: [-120.0 ("y") -120.0 ("y")] -> w375
      frame False {
      }
      frame True {
      }
    }
    n271 = And(x=w356, y=w351) -> (x .and. y?=w350:bool)
    n272 = Less Or Equal?(x=w376, y=w375) -> (x <= y?=w368:bool)
    n273 = Greater Or Equal?(x=w373, y=w374) -> (x >= y?=w371:bool)
    n274 = Less Or Equal?(x=w373, y=w372) -> (x <= y?=w369:bool)
    n275 = Greater Or Equal?(x=w376, y=w377) -> (x >= y?=w370:bool)
    n276 = And(x=w371, y=w370) -> (x .and. y?=w366:bool)
    n277 = Compound Arithmetic op=AND(w355, w369, w368) -> (w367:bool)
    n278 = Or(x=w367, y=w366) -> (x .or. y?=w357:bool)
    n279 = case shown="False" w357 {
      tunnel: [w428 0.0] -> w348
      tunnel: w350 -> [_ _]
      tunnel: w347 -> [w428 _]
      frame False {
      }
      frame True {
        # "makes it relax"
        # "at dart min & at full out or full in \nor at any dart # and fully in"
      }
    }
    n280 = global read "Robot Global Data V.3.0.vi" "Collector Latch"() -> (w359:bool)
    n281 = Select(t=0.0, s=w359, f=w348) -> (s? t:f=w349:dbl)
    n282 = call <vilib>:"WPI_MotorControlSetOutput.vi"("Output"=w349, "MotorControlDevRef"=w395) -> ("Motor Output"=w382:dbl)  [unwired: 7 in, 2 out]
    n283 = global write "Robot Global Data V.3.0.vi" "Collector Speed"(w382) -> ()
    n284 = Wait (ms)(milliseconds to wait=50) -> ()  [unwired: 1 out]
  }
  n285 = call <vilib>:"WPI_MotorControlRefNum Registry Get.vi"("refnum name"="Right Dart Motor") -> ("MotorControlDevRef"=w4:T5)  [unwired: 9 in, 1 out]
  n286 = call <vilib>:"WPI_MotorControlRefNum Registry Get.vi"("refnum name"="Left Dart Motor") -> ("MotorControlDevRef"=w3:T5)  [unwired: 9 in, 1 out]
  n287 = while {
    tunnel: w4 -> [w453]
    tunnel: w3 -> [w452]
    stop <- FALSE stop-if-true
    # "Error correction to keep darts in\nsync plus various other dart \nspeed adjustments"
    n288 = Tick Count (ms)() -> (millisecond timer value=w455:u32)
    n289 = feedback #7() -> (w456:u32)  [unwired: 1 in]
    n290 = feedback-in #7(w455) -> ()
    n291 = Subtract(x=w455, y=w456) -> (x-y=→"Error Loop Run Speed":u32)
    n292 = disable-structure shown="Enabled" {
      disable-tunnel: w453 -> [w460 _]
      disable-tunnel: w452 -> [w459 _]
      frame Enabled {
        w505 = 0.3
        # "This keeps the dart actuators within a reasonable distance of each other"
        # "Rescale error to -1 to 1 scale"
        # "multiply fixes by dart speeds"
        # "change to be max\nallowed inch error"
        n293 = global read "Robot Global Data V.3.0.vi" "# of the Left Dart"() -> (w492:i32)
        n294 = global read "Robot Global Data V.3.0.vi" "# of the Right Dart"() -> (w491:i32)
        n295 = case shown="2" w492 {
          tunnel: [w538 w541 w544 w547] -> w496
          tunnel: [w537 w540 w543 w546] -> w495
          frame 1, Default {
            n296 = global read "Robot Global Data V.3.0.vi" "Dart #1"() -> (w539:T3)
            n297 = Unbundle By Name(w539) -> ("Pot. Voltage"=w538:dbl[], "Corresponding Inches"=w537:dbl[])
          }
          frame 2 {
            n298 = global read "Robot Global Data V.3.0.vi" "Dart #2"() -> (w542:T3)
            n299 = Unbundle By Name(w542) -> ("Pot. Voltage"=w541:dbl[], "Corresponding Inches"=w540:dbl[])
          }
          frame 3 {
            n300 = global read "Robot Global Data V.3.0.vi" "Dart #3"() -> (w545:T3)
            n301 = Unbundle By Name(w545) -> ("Pot. Voltage"=w544:dbl[], "Corresponding Inches"=w543:dbl[])
          }
          frame 4 {
            n302 = global read "Robot Global Data V.3.0.vi" "Dart #4"() -> (w548:T3)
            n303 = Unbundle By Name(w548) -> ("Pot. Voltage"=w547:dbl[], "Corresponding Inches"=w546:dbl[])
          }
        }
        n304 = case shown="3" w491 {
          tunnel: [w526 w529 w532 w535] -> w494
          tunnel: [w525 w528 w531 w534] -> w493
          frame 1, Default {
            n305 = global read "Robot Global Data V.3.0.vi" "Dart #1"() -> (w527:T3)
            n306 = Unbundle By Name(w527) -> ("Pot. Voltage"=w526:dbl[], "Corresponding Inches"=w525:dbl[])
          }
          frame 2 {
            n307 = global read "Robot Global Data V.3.0.vi" "Dart #2"() -> (w530:T3)
            n308 = Unbundle By Name(w530) -> ("Pot. Voltage"=w529:dbl[], "Corresponding Inches"=w528:dbl[])
          }
          frame 3 {
            n309 = global read "Robot Global Data V.3.0.vi" "Dart #3"() -> (w533:T3)
            n310 = Unbundle By Name(w533) -> ("Pot. Voltage"=w532:dbl[], "Corresponding Inches"=w531:dbl[])
          }
          frame 4 {
            n311 = global read "Robot Global Data V.3.0.vi" "Dart #4"() -> (w536:T3)
            n312 = Unbundle By Name(w536) -> ("Pot. Voltage"=w535:dbl[], "Corresponding Inches"=w534:dbl[])
          }
        }
        n313 = global read "Robot Global Data V.3.0.vi" "Right Potentiometer Actual Value"() -> (w498:dbl)
        n314 = global read "Robot Global Data V.3.0.vi" "Left Potentiometer Actual Value"() -> (w499:dbl)
        n315 = Threshold 1D Array(2:w499, 3:w496) -> (0:w510:dbl)  [unwired: 1 in]
        n316 = Threshold 1D Array(2:w498, 3:w494) -> (0:w508:dbl)  [unwired: 1 in]
        n317 = Interpolate 1D Array(1:w510, 2:w495) -> (0:w509:dbl)
        n318 = Interpolate 1D Array(1:w508, 2:w493) -> (0:w497:dbl)
        n319 = Subtract(x=w509, y=w497) -> (x-y=w503:dbl)
        n320 = Negate(x=w505) -> (-x=w506:dbl)
        n321 = Reciprocal(x=w505) -> (1/x=w504:dbl)
        n322 = In Range and Coerce(upper limit=w505, x=w503, lower limit=w506) -> (In Range?=w507:bool)  [unwired: 1 out]
        n323 = Multiply(x=w504, y=w503) -> (x*y=w502:dbl)
        n324 = case shown="False" w507 {
          tunnel: [w549 w576] -> w501
          tunnel: [w550 w578] -> w500
          tunnel: w502 -> [w553 w579]
          frame False {
            # "Darts in completely different positions"
            n325 = Greater?(x=w553, y=1.0) -> (0:w551:bool)
            n326 = case shown="False" w551 {
              tunnel: [w558 w568] -> w550
              tunnel: [w557 w567] -> w549
              frame False {
                # "Right side too far forward"
                n327 = global read "Robot Global Data V.3.0.vi" "Automatic Arms Up and Scale Angle"() -> (w555:bool)
                n328 = global read "Robot Global Data V.3.0.vi" "Left Aux Joystick Y"() -> (w559:dbl)
                n329 = Greater Than 0?(x=w559) -> (x > 0?=w554:bool)
                n330 = Or(x=w554, y=w555) -> (x .or. y?=w556:bool)
                n331 = case shown="False" w556 {
                  tunnel: [0.5 1.0] -> w558
                  tunnel: [1.0 0.5] -> w557
                  frame False {
                  }
                  frame True {
                  }
                }
              }
              frame True {
                # "Left side too far forward"
                n332 = global read "Robot Global Data V.3.0.vi" "Left Aux Joystick Y"() -> (w569:dbl)
                n333 = global read "Robot Global Data V.3.0.vi" "Automatic Arms Up and Scale Angle"() -> (w565:bool)
                n334 = Greater Than 0?(x=w569) -> (x > 0?=w564:bool)
                n335 = Or(x=w564, y=w565) -> (x .or. y?=w566:bool)
                n336 = case shown="False" w566 {
                  tunnel: [1.0 0.5] -> w568
                  tunnel: [0.5 1.0] -> w567
                  frame False {
                  }
                  frame True {
                  }
                }
              }
            }
          }
          frame True {
            n337 = disable-structure shown="Enabled" {
              disable-tunnel: w579 -> [w589 w597]
              disable-tunnel: [w587 w601] -> w577
              disable-tunnel: [w586 w596] -> w575
              disable-tunnel: [w584 w605] -> w574
              frame Disabled {
                w583 = 4.5
                w581 = 1
                w588 = 1.35
                n338 = Subtract(x=w589, y=w588) -> (x-y=w582:dbl)
                n339 = Add(x=w589, y=w588) -> (x+y=w591:dbl)
                n340 = Multiply(x=w582, y=w583) -> (x*y=w594:dbl)
                n341 = Multiply(x=w583, y=w591) -> (x*y=w590:dbl)
                n342 = Divide(x=1, y=w594) -> (x/y=w593:dbl)
                n343 = Divide(x=-1, y=w590) -> (x/y=w580:dbl)
                n344 = Add(x=w593, y=w581) -> (x+y=w587:dbl)
                n345 = global read "Robot Global Data V.3.0.vi" "Left Aux Joystick Y"() -> (w585:dbl)
                n346 = Add(x=w581, y=w580) -> (x+y=w586:dbl)
                n347 = Greater Than 0?(x=w585) -> (x > 0?=w584:bool)
              }
              frame Enabled {
                n348 = Multiply(x=w597, y=-0.1) -> (x*y=w603:dbl)
                n349 = Multiply(x=w597, y=0.1) -> (x*y=w599:dbl)
                n350 = Add(x=w603, y=0.9) -> (x+y=w601:dbl)
                n351 = Add(x=w599, y=0.9) -> (x+y=w596:dbl)
                n352 = global read "Robot Global Data V.3.0.vi" "Left Aux Joystick Y"() -> (w606:dbl)
                n353 = Greater Than 0?(x=w606) -> (x > 0?=w605:bool)
              }
            }
            n354 = case shown="True" w574 {
              tunnel: [w607 w610] -> w578
              tunnel: w577 -> [w608 w610]
              tunnel: [w608 w609] -> w576
              tunnel: w575 -> [w607 w609]
              frame False {
              }
              frame True {
              }
            }
          }
        }
        n355 = global read "Robot Global Data V.3.0.vi" "Right Dart Speed Before Fix"() -> (w475:dbl)
        n356 = global read "Robot Global Data V.3.0.vi" "Left Dart Speed Before Fix"() -> (w488:dbl)
        n357 = global read "Robot Global Data V.3.0.vi" "Right Dart Amps"() -> (w473:dbl)
        n358 = global read "Robot Global Data V.3.0.vi" "Left Dart Amps"() -> (w474:dbl)
        n359 = global write "Robot Global Data V.3.0.vi" "Left Dart Fix"(w500) -> ()
        n360 = global write "Robot Global Data V.3.0.vi" "Right Dart Fix"(w501) -> ()
        n361 = Multiply(x=w501, y=w475) -> (x*y=w489:dbl)
        n362 = Equal To 0?(x=w474) -> (x = 0?=w472:bool)
        n363 = Equal To 0?(x=w473) -> (x = 0?=w471:bool)
        n364 = global read "Robot Global Data V.3.0.vi" "Right Dart Amps"() -> (w479:dbl)
        n365 = global read "Robot Global Data V.3.0.vi" "Left Dart Amps"() -> (w486:dbl)
        n366 = Multiply(x=w488, y=w500) -> (x*y=w490:dbl)
        n367 = disable-structure shown="Enabled" {
          disable-tunnel: w490 -> [w519 w524]
          disable-tunnel: w489 -> [w513 w523]
          disable-tunnel: [w512 w524] -> w483
          disable-tunnel: [w511 w523] -> w466
          frame Disabled {
            n368 = global read "Robot Global Data V.3.0.vi" "Collector Angle Motor Actual Angle"() -> (w516:dbl)
            n369 = global read "Robot Global Data V.3.0.vi" "Collector Angle Motor Actual Angle"() -> (w521:dbl)
            n370 = Less?(x=w516, y=-5) -> (x < y?=w517:bool)
            n371 = Less?(x=w521, y=-5) -> (x < y?=w522:bool)
            n372 = Select(t=w513, s=w517, f=0) -> (s? t:f=w511:dbl)
            n373 = Select(t=w519, s=w522, f=0) -> (s? t:f=w512:dbl)
          }
          frame Enabled {
          }
        }
        n374 = Or(x=w472, y=w471) -> (x .or. y?=w469:bool)
        n375 = Not Equal To 0?(x=w475) -> (x != 0?=w470:bool)
        n376 = And(x=w470, y=w469) -> (x .and. y?=w468:bool)
        n377 = Equal To 0?(x=w479) -> (x = 0?=w477:bool)
        n378 = Equal To 0?(x=w486) -> (x = 0?=w478:bool)
        n379 = Not Equal To 0?(x=w488) -> (x != 0?=w487:bool)
        n380 = Select(t=1.0, s=w468, f=1.0) -> (s? t:f=w465:dbl)
        n381 = Or(x=w478, y=w477) -> (x .or. y?=w476:bool)
        n382 = global read "Robot Global Data V.3.0.vi" "Right Dart Final Speed"() -> (w462:dbl)
        n383 = global read "Robot Global Data V.3.0.vi" "Left Dart Final Speed"() -> (w461:dbl)
        n384 = And(x=w487, y=w476) -> (x .and. y?=w485:bool)
        n385 = Select(t=1.0, s=w485, f=1.0) -> (s? t:f=w481:dbl)
        n386 = Multiply(x=w466, y=w465) -> (x*y=w467:dbl)
        n387 = Multiply(x=w481, y=w483) -> (x*y=w484:dbl)
        n388 = global write "Robot Global Data V.3.0.vi" "Right Dart Final Speed"(w467) -> ()
        n389 = call <vilib>:"WPI_MotorControlSetOutput.vi"("Output"=w461, "MotorControlDevRef"=w459) -> ()  [unwired: 7 in, 3 out]
        n390 = call <vilib>:"WPI_MotorControlSetOutput.vi"("Output"=w462, "MotorControlDevRef"=w460) -> ()  [unwired: 7 in, 3 out]
        n391 = global write "Robot Global Data V.3.0.vi" "Left Dart Final Speed"(w484) -> ()
      }
      frame Disabled {
        n392 = global read "Robot Global Data V.3.0.vi" "Left Dart Speed Before Fix"() -> (w611:dbl)
        n393 = global read "Robot Global Data V.3.0.vi" "Right Dart Speed Before Fix"() -> (w612:dbl)
        n394 = global write "Robot Global Data V.3.0.vi" "Left Dart Final Speed"(w611) -> ()
        n395 = global write "Robot Global Data V.3.0.vi" "Right Dart Final Speed"(w612) -> ()
      }
    }
    n396 = Wait (ms)(milliseconds to wait=50) -> ()  [unwired: 1 out]
  }
